vi "LINC Format Format String.vi"(10 "format in":string) -> (2 "format out":string)   [LabVIEW 2018, in "STEPkgDriver_LINC.lvlib"]
uses:
  STEPkgDriver_LINC.lvlib
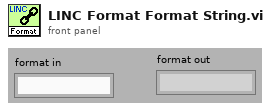
[diagram p1: front panel]
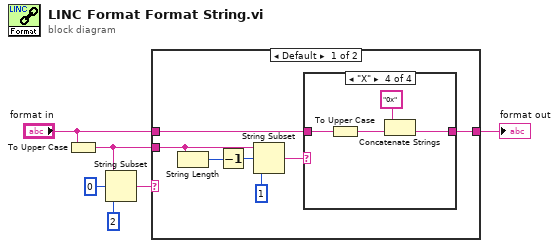
[diagram p0: block diagram]
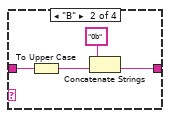
[diagram p3: hidden frame]
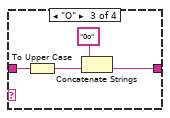
[diagram p4: hidden frame]
diagram:
  n1 = To Upper Case(1:"format in") -> (0:w2:string)
  n2 = String Subset(string=w2, offset (0)=0, length (rest)=2 ("length (rest)")) -> (substring=w3:string)
  n3 = case shown="Default" w3 {
    tunnel: [w10 w27] -> w6
    tunnel: "format in" -> [w8 w27]
    tunnel: w2 -> [w7 _]
    frame Default {
      n4 = String Length(string=w7) -> (length=w13:i32)
      n5 = Decrement(x=w13) -> (x-1=w12:i32)
      n6 = String Subset(string=w7, offset (0)=w12, length (rest)=1 ("length (rest)")) -> (substring=w9:string)
      n7 = case shown="\"X\"" w9 {
        tunnel: w8 -> [w14 w18 w22 w26]
        tunnel: [w14 w17 w21 w25] -> w10
        frame Default {
        }
        frame "B" {
          n8 = To Upper Case(1:w18) -> (0:w15:string)
          n9 = Concatenate Strings("0b", w15) -> (w17:string)
        }
        frame "O" {
          n10 = To Upper Case(1:w22) -> (0:w19:string)
          n11 = Concatenate Strings("0o", w19) -> (w21:string)
        }
        frame "X" {
          n12 = To Upper Case(1:w26) -> (0:w23:string)
          n13 = Concatenate Strings("0x", w23) -> (w25:string)
        }
      }
    }
    frame "0B", "0O", "0X" {
    }
  }
  "format out" <- w6
